vi "DtOLTimingSetOutput.vi"(7 "Sample Mode":T1(ring)=enum."Resend One Buffer", 8 "error in (no error)":errorcluster, 9 "Timing":T2(ring), 10 "Sample Freq (Hz)":dbl=1000.0, 11 "Task in":i32) -> (0 "error out":errorcluster, 2 "Actual Sample Freq":dbl, 3 "Task out":i32)   [LabVIEW 2022 SP3]
doc: "Specifies all of the timing and buffer related details when streaming output data."
uses:
  DtLvLink.lvlib
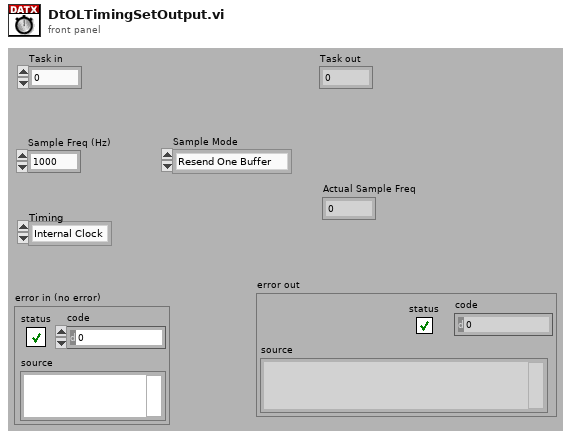
[diagram p1: front panel]
types:
  T1 = enum32{"Finite", "Continuous", "Resend One Buffer"}
  T2 = enum32{"Internal Clock", "External Clock", "No Timing"}
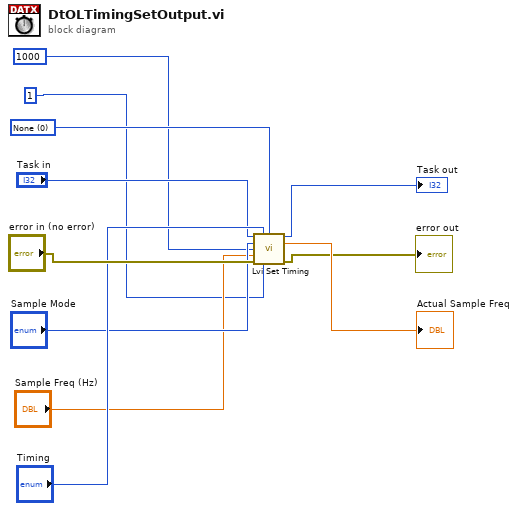
[diagram p0: block diagram]
diagram:
  w7 = 0 items=["None", "Master", "Slave"] ("SynchronizationModes SyncMode")
  n1 = call "Lvi Set Timing.vi"("TaskRef"="Task in", "ClkSource"="Timing", "SyncMode"=w7, "SampleMode"="Sample Mode", "PointsPerChan"=u32 1000 ("Int32 PointsPerChan"), "SampleRate"="Sample Freq (Hz)", "error in (no error)"="error in (no error)", "NumBuffers"=u32 1 ("Int32 NumBuffers")) -> ("TaskRef out"=→"Task out":i32, "ActualSampleRate"=→"Actual Sample Freq":dbl, "error out"=→"error out":errorcluster)  [unwired: 4 in, 1 out]
